vi "He3ReadOut.vi"(7 "stop_external":refnum<vi>, 10 "status_ref":refnum<vi>, 11 "pressure_ref":refnum<vi>) -> ()   [LabVIEW 2019]
uses:
  <vilib>/Instr/_visa.llb/VISA Flush IO Buffer Mask.ctl
  <vilib>/Instr/_visa.llb/VISA Configure Serial Port (Instr).vi
  Global 1.vi
panel:
  in  "VISA":refnum<visa-resource-name>="COM16"
  out "status string":string
  out "Array":bool[](array[boolean])
  out "Error at VISA Read 6":errorcluster
  out "Error at segmenting output 5":errorcluster
  out "MKS 670 Status":bool
  out "Read buffer":string
  in  "Pressure (Torr)":dbl
  in  "stop":bool
  out "He3 Sensor":dbl
  out "Waveform Chart 2":dbl(graph)
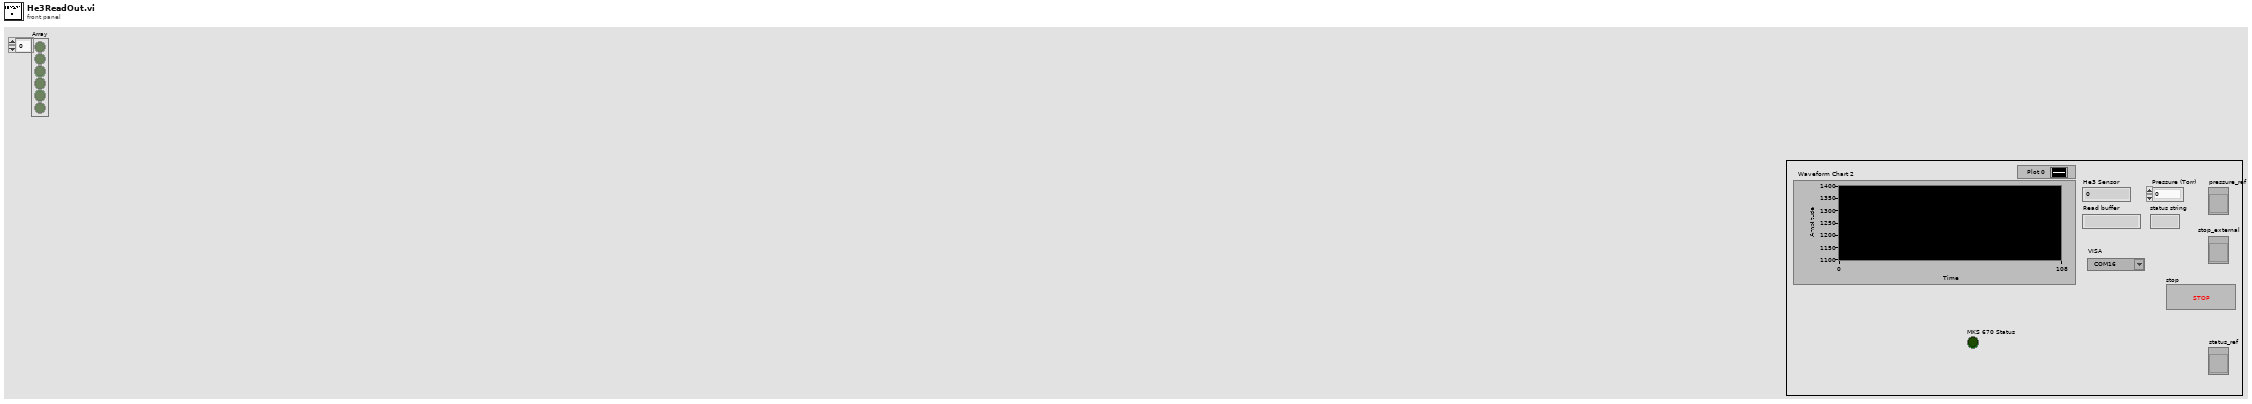
[diagram p1: front panel]
types:
  T1 = typedef "VISA Flush IO Buffer Mask.ctl" = u16
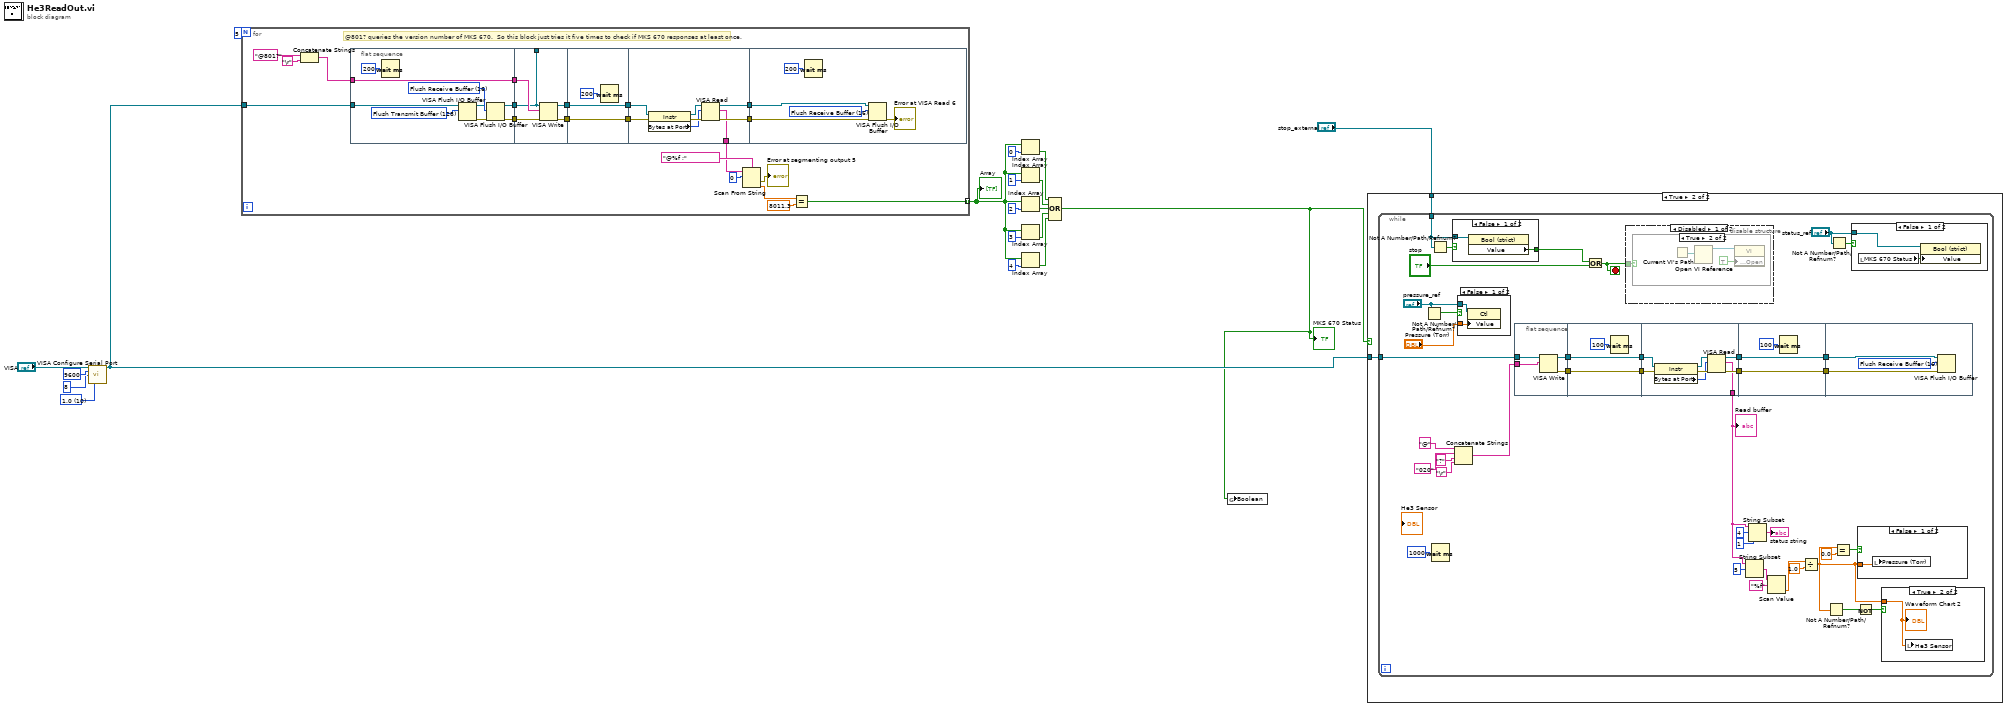
[diagram p0: block diagram]
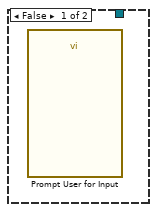
[diagram p2: hidden frame]
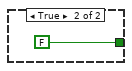
[diagram p7: hidden frame]
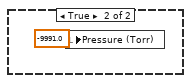
[diagram p8: hidden frame]
diagram:
  w19 = u16 10 items=["1.0"=10, "1.5"=15, "2.0"=20] ("stop bits (10: 1 bit)")
  n1 = call-poly "VISA Configure Serial Port"("VISA resource name"="VISA", "baud rate (9600)"=u32 9600, "data bits (8)"=u16 8, "stop bits (10: 1 bit)"=w19) -> ("VISA resource name out"=w4:refnum<visa-resource-name>)  [unwired: 10 in, 1 out]
  n2 = for {
    N: 5 -> [_]
    tunnel: w4 -> [w24]
    tunnel: [w23] -> w5 mode=indexing
    # "@801? queries the version number of MKS 670.  So this block just tries it five times to check if MKS 670 responses at least once."
    n3 = Concatenate Strings("@801?" ("string"), "\r") -> (w20:string)
    n4 = flat-sequence {
      tunnel: w24 -> [w43]
      tunnel: w20 -> [w48]
      tunnel: [w48] -> w39
      tunnel: [w42] -> w38
      tunnel: [w41] -> w37
      tunnel: [w50] -> _
      tunnel: [w52] -> w36
      tunnel: [w51] -> w35
      tunnel: w39 -> [w53]
      tunnel: w38 -> [w50]
      tunnel: w37 -> [w49]
      tunnel: w36 -> [w55]
      tunnel: [w55] -> w34
      tunnel: w35 -> [w54]
      tunnel: [w54] -> w33
      tunnel: w34 -> [w61]
      tunnel: w33 -> [w60]
      tunnel: [w59] -> w32
      tunnel: [w58] -> w31
      tunnel: [w57] -> w25
      tunnel: w32 -> [w68]
      tunnel: w31 -> [w67]
      frame #0 {
        w47 = T1 16 items=["Flush Receive Buffer"=16, "Write Transmit Buffer to Device"=32, "Flush Receive Buffer (No I/O)"=64, "Flush Transmit Buffer"=128] ("Mask")
        w44 = T1 128 items=["Flush Receive Buffer"=16, "Write Transmit Buffer to Device"=32, "Flush Receive Buffer (No I/O)"=64, "Flush Transmit Buffer"=128] ("Mask")
        n5 = Wait (ms)(milliseconds to wait=u32 200) -> ()  [unwired: 1 out]
        n6 = VISA Flush I/O Buffer(VISA resource name=w43, mask (16)=w44) -> (VISA resource name out=w45:refnum<visa-resource-name>, error out=w46:errorcluster)  [unwired: 1 in]
        n7 = VISA Flush I/O Buffer(VISA resource name=w45, mask (16)=w47, error in (no error)=w46) -> (VISA resource name out=w42:refnum<visa-resource-name>, error out=w41:errorcluster)
      }
      frame #1 {
        n8 = VISA Write(VISA resource name=w50, write buffer=w53, error in (no error)=w49) -> (VISA resource name out=w52:refnum<visa-resource-name>, error out=w51:errorcluster)  [unwired: 1 out]
      }
      frame #2 {
        n9 = Wait (ms)(milliseconds to wait=u32 200) -> ()  [unwired: 1 out]
      }
      frame #3 {
        n10 = property class="Instr"(reference=w61, error in=w60) -> (reference out=w62:refnum<visa-resource-name>, error out=w64:errorcluster, "Bytes at Port"=w63:u32)
        n11 = VISA Read(VISA resource name=w62, byte count=w63, error in (no error)=w64) -> (VISA resource name out=w59:refnum<visa-resource-name>, read buffer=w57:string, error out=w58:errorcluster)  [unwired: 1 out]
      }
      frame #4 {
        w65 = T1 16 items=["Flush Receive Buffer"=16, "Write Transmit Buffer to Device"=32, "Flush Receive Buffer (No I/O)"=64, "Flush Transmit Buffer"=128] ("Mask")
        n12 = Wait (ms)(milliseconds to wait=u32 200) -> ()  [unwired: 1 out]
        n13 = VISA Flush I/O Buffer(VISA resource name=w68, mask (16)=w65, error in (no error)=w67) -> (error out=→"Error at VISA Read 6":errorcluster)  [unwired: 1 out]
      }
    }
    n14 = Scan From String(format string="@%f ;", input string=w25, initial scan location=u32 0) -> (error out=→"Error at segmenting output 5":errorcluster, output 1=w27:dbl)  [unwired: 2 in, 2 out]
    n15 = Equal?(x=w27, y=8011.3) -> (x = y?=w23:bool)
  }
  "Array" <- w5
  n16 = Index Array(array=w5, index=0) -> (element=w9:bool)
  n17 = Index Array(array=w5, index=1) -> (element=w10:bool)
  n18 = Index Array(array=w5, index=2) -> (element=w8:bool)
  n19 = Index Array(array=w5, index=3) -> (element=w7:bool)
  n20 = Index Array(array=w5, index=4) -> (element=w6:bool)
  n21 = Compound Arithmetic op=OR(w9, w10, w8, w7, w6) -> (w3:bool)
  "MKS 670 Status" <- w3
  n22 = global write "Global 1.vi" "Boolean"(w3) -> ()
  n23 = case shown="True" w3 {
    tunnel: w4 -> [_ w71]
    tunnel: "stop_external" -> [_ w70]
    frame False {
      n24 = call "Prompt User for Input"() -> ()  [unwired: 18 in, 2 out]
    }
    frame True {
      n25 = while {
        tunnel: w71 -> [w90]
        tunnel: w70 -> [w77]
        stop <- w80 stop-if-true
        n26 = Not A Number/Path/Refnum?(number/path/refnum="pressure_ref") -> (NaN/Path/Refnum?=w72:bool)
        n27 = Not A Number/Path/Refnum?(number/path/refnum=w77) -> (NaN/Path/Refnum?=w81:bool)
        n28 = Wait (ms)(milliseconds to wait=u32 1000) -> ()  [unwired: 1 out]
        n29 = case shown="False" w81 {
          tunnel: [w119 FALSE] -> w78
          tunnel: w77 -> [w120 _]
          frame False {
            n30 = property class="Bool (strict)"(reference=w120) -> ("Value"=w119:bool)  [unwired: 1 in, 2 out]
          }
          frame True {
          }
        }
        n31 = Concatenate Strings("@" ("string"), "020" ("string"), "?" ("string"), "\r") -> (w95:string)
        n32 = case shown="False" w72 {
          tunnel: "pressure_ref" -> [w116 _]
          tunnel: "Pressure (Torr)" -> [w115 _]
          frame False {
            n33 = property class="Ctl"(reference=w116, "Value"=w115) -> ()  [unwired: 1 in, 2 out]
          }
          frame True {
          }
        }
        n34 = flat-sequence {
          tunnel: w95 -> [w125]
          tunnel: w90 -> [w124]
          tunnel: [w123] -> w99
          tunnel: [w122] -> w98
          tunnel: w99 -> [w127]
          tunnel: [w127] -> w97
          tunnel: w98 -> [w126]
          tunnel: [w126] -> w96
          tunnel: w97 -> [w133]
          tunnel: w96 -> [w132]
          tunnel: [w131] -> w94
          tunnel: [w130] -> w93
          tunnel: [w129] -> w85
          tunnel: w94 -> [w139]
          tunnel: w93 -> [w138]
          tunnel: [w139] -> w92
          tunnel: [w138] -> w91
          tunnel: w92 -> [w142]
          tunnel: w91 -> [w141]
          frame #0 {
            n35 = VISA Write(VISA resource name=w124, write buffer=w125) -> (VISA resource name out=w123:refnum<visa-resource-name>, error out=w122:errorcluster)  [unwired: 1 in, 1 out]
          }
          frame #1 {
            n36 = Wait (ms)(milliseconds to wait=u32 100) -> ()  [unwired: 1 out]
          }
          frame #2 {
            n37 = property class="Instr"(reference=w133, error in=w132) -> (reference out=w134:refnum<visa-resource-name>, error out=w136:errorcluster, "Bytes at Port"=w135:u32)
            n38 = VISA Read(VISA resource name=w134, byte count=w135, error in (no error)=w136) -> (VISA resource name out=w131:refnum<visa-resource-name>, read buffer=w129:string, error out=w130:errorcluster)  [unwired: 1 out]
          }
          frame #3 {
            n39 = Wait (ms)(milliseconds to wait=u32 100) -> ()  [unwired: 1 out]
          }
          frame #4 {
            w140 = T1 16 items=["Flush Receive Buffer"=16, "Write Transmit Buffer to Device"=32, "Flush Receive Buffer (No I/O)"=64, "Flush Transmit Buffer"=128] ("Mask")
            n40 = VISA Flush I/O Buffer(VISA resource name=w142, mask (16)=w140, error in (no error)=w141) -> ()  [unwired: 2 out]
          }
        }
        n41 = Or(x=w78, y="stop") -> (x .or. y?=w80:bool)
        n42 = disable-structure shown="Disabled" {
          disable-tunnel: w80 -> [w111 _]
          frame Disabled {
            n43 = case shown="True" w111 {
              frame False {
              }
              frame True {
                n44 = Current VI's Path() -> (path=w114:path)
                n45 = Open VI Reference(vi path=w114) -> (vi reference=w113:refnum<vi>)  [unwired: 5 in, 1 out]
                n46 = property class="VI"(reference=w113, "Front Panel Window:Open"=TRUE) -> ()  [unwired: 1 in, 2 out]
              }
            }
          }
          frame Enabled {
          }
        }
        n47 = String Subset(string=w85, offset (0)=5) -> (substring=w84:string)  [unwired: 1 in]
        n48 = String Subset(string=w85, offset (0)=4, length (rest)=1 ("length (rest)")) -> (substring=→"status string":string)
        n49 = Scan Value(string=w84, format string="%f") -> (value=w82:dbl)  [unwired: 1 in, 1 out]
        n50 = Divide(x=w82, y=1.0) -> (x/y=w100:dbl)
        n51 = Not A Number/Path/Refnum?(number/path/refnum=w100) -> (NaN/Path/Refnum?=w107:bool)
        n52 = Not A Number/Path/Refnum?(number/path/refnum="status_ref") -> (NaN/Path/Refnum?=w76:bool)
        n53 = Equal?(x=w100, y=0.0) -> (x = y?=w101:bool)
        n54 = case shown="False" w76 {
          tunnel: "status_ref" -> [w117 _]
          frame False {
            n55 = local read "MKS 670 Status"() -> (w118:bool)
            n56 = property class="Bool (strict)"(reference=w117, "Value"=w118) -> ()  [unwired: 1 in, 2 out]
          }
          frame True {
          }
        }
        n57 = Not(x=w107) -> (.not. x?=w106:bool)
        n58 = case shown="False" w101 {
          tunnel: w100 -> [w143 _]
          frame False {
            n59 = local write "Pressure (Torr)"(w143) -> ()
          }
          frame True {
            n60 = local write "Pressure (Torr)"(-9991.0 ("Numeric")) -> ()
          }
        }
        n61 = case shown="True" w106 {
          tunnel: w100 -> [_ w145]
          frame False {
          }
          frame True {
            n62 = local write "He3 Sensor"(w145) -> ()
            "Waveform Chart 2" <- w145
          }
        }
        "Read buffer" <- w85
      }
    }
  }
